vi "校准参数转data(子VI).vi"(10 "改变?":bool, 11 "校准信息":T1) -> (3 "数组":string[][](array[string]))   [LabVIEW 2016, in "数据传输系统-02.lvlib"]
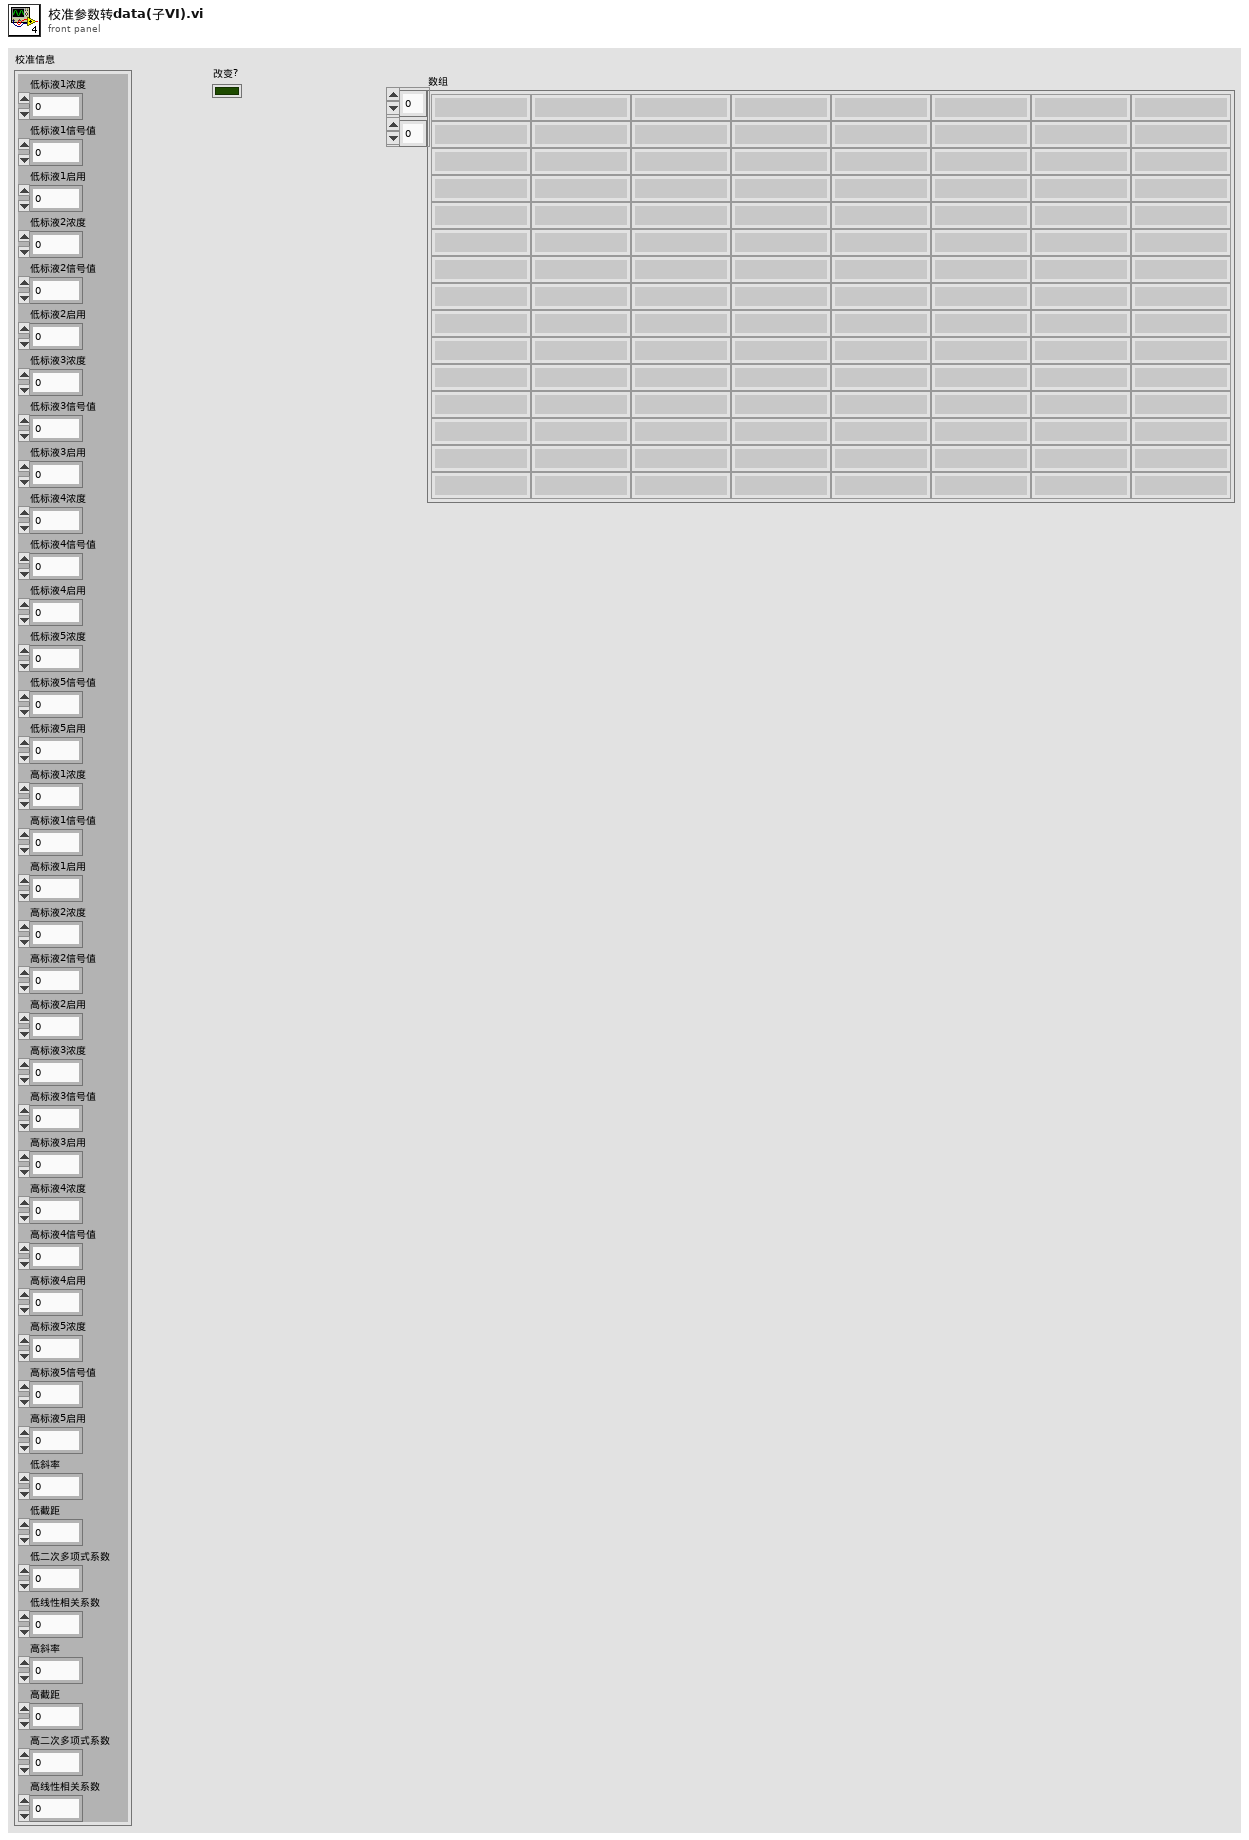
[diagram p1: front panel]
types:
  T1 = cluster{"低标液1浓度":dbl, "低标液1信号值":dbl, "低标液1启用":u16, "低标液2浓度":dbl, "低标液2信号值":dbl, "低标液2启用":u16, "低标液3浓度":dbl, "低标液3信号值":dbl, "低标液3启用":u16, "低标液4浓度":dbl, "低标液4信号值":dbl, "低标液4启用":u16, "低标液5浓度":dbl, "低标液5信号值":dbl, "低标液5启用":u16, "高标液1浓度":dbl, "高标液1信号值":dbl, "高标液1启用":u16, "高标液2浓度":dbl, "高标液2信号值":dbl, "高标液2启用":u16, "高标液3浓度":dbl, "高标液3信号值":dbl, "高标液3启用":u16, "高标液4浓度":dbl, "高标液4信号值":dbl, "高标液4启用":u16, "高标液5浓度":dbl, "高标液5信号值":dbl, "高标液5启用":u16, "低斜率":dbl, "低截距":dbl, "低二次多项式系数":dbl, "低线性相关系数":dbl, "高斜率":dbl, "高截距":dbl, "高二次多项式系数":dbl, "高线性相关系数":dbl}
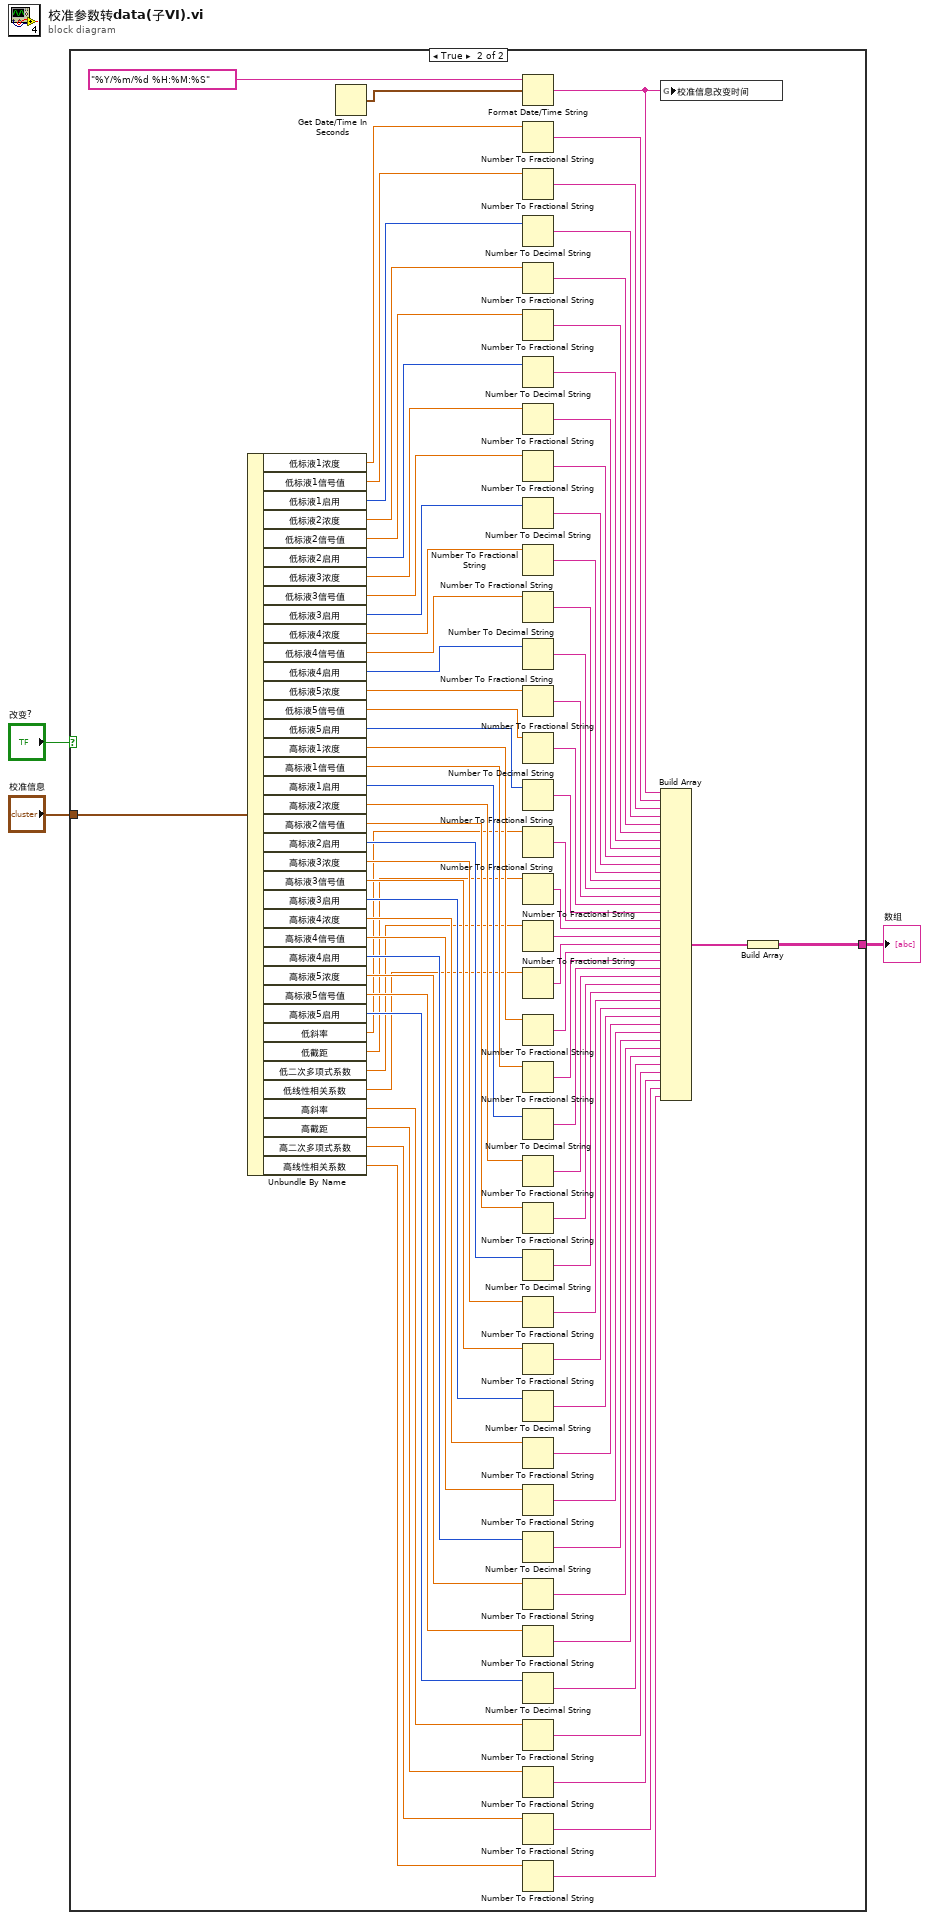
[diagram p0: block diagram]
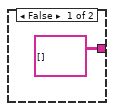
[diagram p2: hidden frame]
diagram:
  n1 = case shown="True" "改变?" {
    tunnel: [string[][] [] w86] -> w3
    tunnel: "校准信息" -> [_ w62]
    frame False {
    }
    frame True {
      n2 = Unbundle By Name(w62) -> ("低标液1浓度"=w63:dbl, "低标液1信号值"=w67:dbl, "低标液1启用"=w69:u16, "低标液2浓度"=w71:dbl, "低标液2信号值"=w73:dbl, "低标液2启用"=w61:u16, "低标液3浓度"=w75:dbl, "低标液3信号值"=w76:dbl, "低标液3启用"=w59:u16, "低标液4浓度"=w77:dbl, "低标液4信号值"=w78:dbl, "低标液4启用"=w57:u16, "低标液5浓度"=w55:dbl, "低标液5信号值"=w79:dbl, "低标液5启用"=w53:u16, "高标液1浓度"=w51:dbl, "高标液1信号值"=w50:dbl, "高标液1启用"=w49:u16, "高标液2浓度"=w47:dbl, "高标液2信号值"=w46:dbl, "高标液2启用"=w45:u16, "高标液3浓度"=w41:dbl, "高标液3信号值"=w40:dbl, "高标液3启用"=w39:u16, "高标液4浓度"=w38:dbl, "高标液4信号值"=w37:dbl, "高标液4启用"=w36:u16, "高标液5浓度"=w35:dbl, "高标液5信号值"=w34:dbl, "高标液5启用"=w33:u16, "低斜率"=w22:dbl, "低截距"=w21:dbl, "低二次多项式系数"=w20:dbl, "低线性相关系数"=w19:dbl, "高斜率"=w14:dbl, "高截距"=w13:dbl, "高二次多项式系数"=w12:dbl, "高线性相关系数"=w11:dbl)
      n3 = Get Date/Time In Seconds() -> (seconds since 1Jan1904=w65:timestamp)
      n4 = Format Date/Time String(time format string (%c)="%Y/%m/%d %H:%M:%S" ("时间格式字符串(%c)"), seconds (now)=w65) -> (date/time string=w23:string)  [unwired: 1 in]
      n5 = Number To Fractional String(number=w63) -> (F-format string=w66:string)  [unwired: 3 in]
      n6 = Number To Fractional String(number=w67) -> (F-format string=w68:string)  [unwired: 3 in]
      n7 = Number To Decimal String(number=w69) -> (decimal integer string=w70:string)  [unwired: 1 in]
      n8 = Number To Fractional String(number=w71) -> (F-format string=w72:string)  [unwired: 3 in]
      n9 = Number To Fractional String(number=w73) -> (F-format string=w74:string)  [unwired: 3 in]
      n10 = Number To Decimal String(number=w61) -> (decimal integer string=w60:string)  [unwired: 1 in]
      n11 = Number To Fractional String(number=w75) -> (F-format string=w80:string)  [unwired: 3 in]
      n12 = Number To Fractional String(number=w76) -> (F-format string=w81:string)  [unwired: 3 in]
      n13 = Number To Decimal String(number=w59) -> (decimal integer string=w58:string)  [unwired: 1 in]
      n14 = Number To Fractional String(number=w77) -> (F-format string=w82:string)  [unwired: 3 in]
      n15 = Number To Fractional String(number=w78) -> (F-format string=w83:string)  [unwired: 3 in]
      n16 = Number To Decimal String(number=w57) -> (decimal integer string=w56:string)  [unwired: 1 in]
      n17 = Number To Fractional String(number=w55) -> (F-format string=w54:string)  [unwired: 3 in]
      n18 = Number To Fractional String(number=w79) -> (F-format string=w84:string)  [unwired: 3 in]
      n19 = Number To Decimal String(number=w53) -> (decimal integer string=w52:string)  [unwired: 1 in]
      n20 = Number To Fractional String(number=w22) -> (F-format string=w18:string)  [unwired: 3 in]
      n21 = Number To Fractional String(number=w21) -> (F-format string=w17:string)  [unwired: 3 in]
      n22 = Number To Fractional String(number=w20) -> (F-format string=w16:string)  [unwired: 3 in]
      n23 = Number To Fractional String(number=w19) -> (F-format string=w15:string)  [unwired: 3 in]
      n24 = Number To Fractional String(number=w51) -> (F-format string=w5:string)  [unwired: 3 in]
      n25 = Number To Fractional String(number=w50) -> (F-format string=w6:string)  [unwired: 3 in]
      n26 = Number To Decimal String(number=w49) -> (decimal integer string=w48:string)  [unwired: 1 in]
      n27 = Number To Fractional String(number=w47) -> (F-format string=w44:string)  [unwired: 3 in]
      n28 = Number To Fractional String(number=w46) -> (F-format string=w43:string)  [unwired: 3 in]
      n29 = Number To Decimal String(number=w45) -> (decimal integer string=w42:string)  [unwired: 1 in]
      n30 = Number To Fractional String(number=w41) -> (F-format string=w32:string)  [unwired: 3 in]
      n31 = Number To Fractional String(number=w40) -> (F-format string=w31:string)  [unwired: 3 in]
      n32 = Number To Decimal String(number=w39) -> (decimal integer string=w30:string)  [unwired: 1 in]
      n33 = Number To Fractional String(number=w38) -> (F-format string=w29:string)  [unwired: 3 in]
      n34 = Number To Fractional String(number=w37) -> (F-format string=w28:string)  [unwired: 3 in]
      n35 = Number To Decimal String(number=w36) -> (decimal integer string=w27:string)  [unwired: 1 in]
      n36 = Number To Fractional String(number=w35) -> (F-format string=w26:string)  [unwired: 3 in]
      n37 = Number To Fractional String(number=w34) -> (F-format string=w25:string)  [unwired: 3 in]
      n38 = Number To Decimal String(number=w33) -> (decimal integer string=w24:string)  [unwired: 1 in]
      n39 = Number To Fractional String(number=w14) -> (F-format string=w10:string)  [unwired: 3 in]
      n40 = Number To Fractional String(number=w13) -> (F-format string=w9:string)  [unwired: 3 in]
      n41 = Number To Fractional String(number=w12) -> (F-format string=w8:string)  [unwired: 3 in]
      n42 = Number To Fractional String(number=w11) -> (F-format string=w7:string)  [unwired: 3 in]
      n43 = global write "全局1.vi" "校准信息改变时间"(w23) -> ()
      n44 = Build Array(w23, w66, w68, w70, w72, w74, w60, w80, w81, w58, w82, w83, w56, w54, w84, w52, w18, w17, w16, w15, w5, w6, w48, w44, w43, w42, w32, w31, w30, w29, w28, w27, w26, w25, w24, w10, w9, w8, w7) -> (w85:string[])
      n45 = Build Array(w85) -> (w86:string[][])
    }
  }
  "数组" <- w3
